vi "PH_Cont-601k_PowerUnit.SM PSU condition check.vi"(0 "VI in":refnum<vi>, 2 "Wanted Device Mode (READY)":T2=enum."READY", 3 "Wanted Device Readyness (OPERATING)":T1=enum."OPERATING", 5 "error in (no error)":errorcluster) -> (14 "VI out":refnum<vi>, 17 "Condition fullfilled":bool, 19 "error out":errorcluster)   [LabVIEW 2014, in "PH_Cont-601k_PowerUnit.lvlib"]
uses:
  PH_Cont-601k_PowerUnit.lvlib
  PH_Devices/PH_Cont-601k_PSU/PH_Cont-601k_PSU.Mode.ctl
  PH_Devices/PH_Cont-601k_PSU/PH_Cont-601k_PSU.Readyness Device.ctl
  PH_Devices/PH_Cont-601k_PSU/PH_Cont-601k_PSU.Configuration.ctl
  PH_Devices/PH_Cont-601k_PSU/PH_Cont-601k_PSU.Readyness Program.ctl
  PH_Devices/PH_Cont-601k_PSU/PH_Cont-601k_PSU.lvlib
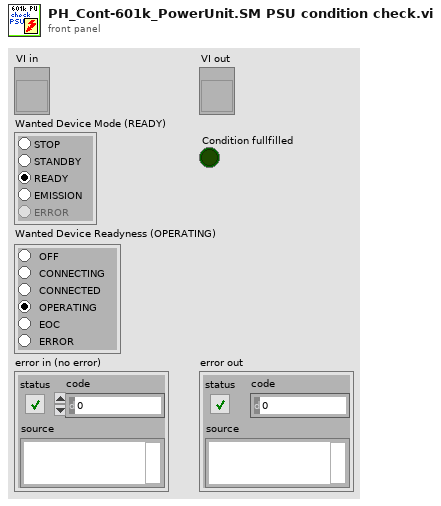
[diagram p1: front panel]
types:
  T1 = typedef "PH_Cont-601k_PSU.lvlib/PH_Cont-601k_PSU.Readyness Device.ctl" = enum32{"OFF", "CONNECTING", "CONNECTED", "OPERATING", "EOC", "ERROR"}
  T2 = typedef "PH_Cont-601k_PSU.lvlib/PH_Cont-601k_PSU.Mode.ctl" = enum32{"STOP", "STANDBY", "READY", "EMISSION", "ERROR"}
  T3 = typedef "PH_Cont-601k_PSU.lvlib/PH_Cont-601k_PSU.Readyness Program.ctl" = enum32{"OFF", "POWER", "INTERLOCK"}
  T4 = typedef "PH_Cont-601k_PSU.lvlib/PH_Cont-601k_PSU.Configuration.ctl" = u16
  T5 = typedef "PH_Cont-601k_PSU.lvlib/PH_Cont-601k_PSU.i attribute.ctl" = cluster{"GUI Refs":T6, "Interlock":bool, "Service ID applied Voltage":i32, "Device Settings":cluster{"Configuration":T4, "Flash Interval [s]":dbl, "Mode":T2, "Voltage [V]":u16, "Charge":bool, "VISA resource name":refnum<visa-resource-name>}, "Readyness":T7, "Information":cluster{"VISA resource name":refnum<visa-resource-name>, "Tagname Power On":string, "Interlock":cluster{"Instance":string, "Tagname":string}, "Limits [V]":cluster{"Lower":dbl, "Upper":dbl}, "Tagname PSU On":string}, "R2S":bool, "Charge is allowed":bool}
  T6 = typedef "PH_Cont-601k_PSU.lvlib/PH_Cont-601k_PSU.GUI Refs.ctl" = cluster{"Power On":refnum<vi>, "Hard- and Software":refnum<vi>, "Device Status":refnum<vi>, "Device Error":refnum<vi>, "Configuration":refnum<vi>, "Flash Interval [s]":refnum<vi>, "Interlock":refnum<vi>, "Interlock Indicator":refnum<vi>, "Voltage [V]":refnum<vi>, "Readyness":refnum<vi>, "Mode":refnum<vi>, "Reset Error":refnum<vi>, "Expert working":refnum<vi>, "Charge":refnum<vi>, "PSU On":refnum<vi>}
  T7 = typedef "PH_Cont-601k_PSU.lvlib/PH_Cont-601k_PSU.Readyness.ctl" = cluster{"Program":T3, "Device":T1}
  T8 = cluster{"Program":T3, "Wanted Device Readyness (OPERATING)":T1}
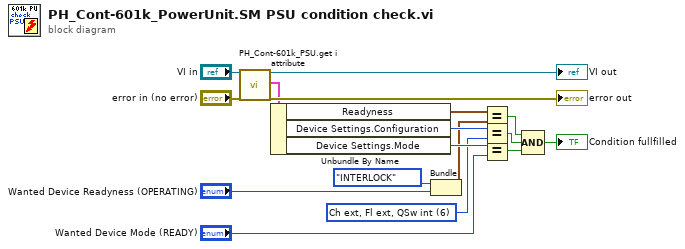
[diagram p0: block diagram]
diagram:
  w6 = T4 6 items=["Ch intl, Fl intl, QSw intl", "Ch intl, Fl intl, QSw ext", "Ch intl, Fl ext, QSw intl", "Ch intl, Fl ext, QSw ext", "Ch ext, Fl int, QSw int", "Ch ext, Fl int, QSw ext", "Ch ext, Fl ext, QSw int", "Ch ext, Fl ext, QSw ext"] ("y")
  n1 = call "PH_Cont-601k_PSU.get i attribute.vi"("i ref in"="VI in", "error in (no error)"="error in (no error)") -> ("i ref out"=→"VI out":refnum<vi>, "i attribute"=w10:T5, "error out"=→"error out":errorcluster)  [unwired: 15 in]
  n2 = Unbundle By Name(w10) -> ("Readyness"=w9:T7, "Device Settings.Configuration"=w8:T4, "Device Settings.Mode"=w7:T2)
  n3 = Bundle("Program"=PH_Cont-601k_PSU.Readyness_Program."INTERLOCK", "Wanted Device Readyness (OPERATING)"="Wanted Device Readyness (OPERATING)") -> (w1:T8)  [unwired: 1 in]
  n4 = Equal?(x=w9, y=w1) -> (x = y?=w5:bool)
  n5 = Equal?(x=w8, y=w6) -> (x = y?=w4:bool)
  n6 = Equal?(x=w7, y="Wanted Device Mode (READY)") -> (x = y?=w12:bool)
  n7 = Compound Arithmetic op=AND(w5, w4, w12) -> (→"Condition fullfilled":bool)
